vi "6812B_AC_old.vi"() -> ()   [LabVIEW 2019]
doc: "Shows how to generate a standard output."
uses:
  <instrlib>/Agilent 681x Series/Public/Data/Read Single Measurement (Current).vi
  <instrlib>/Agilent 681x Series/Agilent 681x Series.lvlib
panel:
  out "Flag":bool
  in  "Maximum Time (10000 ms)":i32=10000
  in  "Sense Source (0: Internal)":u16(ring) items=["Internal", "External"]
  in  "Sample Spacing (25 us)":dbl=2.5e-05 format="%^.2g"
  in  "Relative Trigger Samples (0)":i32
  out "Peak Current":dbl
  out "AC + DC RMS Current":dbl
  out "AC RMS Current":dbl
  out "DC Current":dbl
  in  "Pulse Characteristic Value (%)":dbl=50.0 format="%#.4g"
  in  "Pulse Characteristic (0: Duty Cycle)":u16(ring) items=["Duty Cycle", "Pulse Width"]
  in  "Period (s)":dbl=0.03333 format="%#.4g"
  in  "Trigger Delay (s)":dbl format="%#.5g"
  in  "Pulse Count":dbl=1.0 format="%#.4g"
  in  "Voltage Mode (0: Fix)":u16(ring) items=["Fixed", "Step", "Pulse", "List"]
  in  "Triggered Voltage Amplitude (V)":dbl=1.0 format="%#.4g"
  in  "Parar":bool
  in  "Peak Current Limit (13 A)":dbl=13.0 format="%#.4g"
  in  "RMS Current Limit (1 A)":dbl=1.0 format="%#.4g"
  in  "Voltage Amplitude (1.0 V)":dbl=1.0 format="%#.4g"
  in  "Output Frequency (60 Hz)":dbl=60.0 format="%#.4g"
  in  "Output Waveform Type (0: Sinusoid)":u16(ring) items=["Sinusoid", "Square", "Clipped Sinusoid", "User Specified"]
  in  "Serial Configuration":T1={"Baud Rate"=9600, "Parity"=0, "Data Bits"=8} {"Data Bits" items=["7"=7, "8"=8]; "Parity" items=["None", "Odd", "Even", "Mark", "Space"]; "Baud Rate" items=["300"=300, "600"=600, "1200"=1200, "2400"=2400, "4800"=4800, "9600"=9600]}
  in  "VISA resource name":refnum<visa-resource-name>
  # "(c) 2008-2021 National Instruments Corp.  ALL RIGHTS RESERVED."
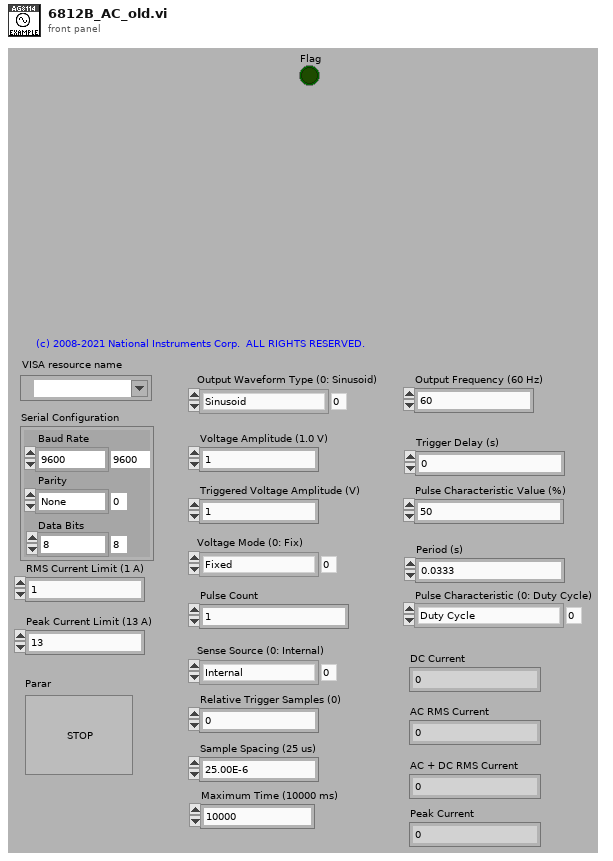
[diagram p1: front panel]
types:
  T1 = cluster{"Baud Rate":u32, "Parity":u16, "Data Bits":u16}
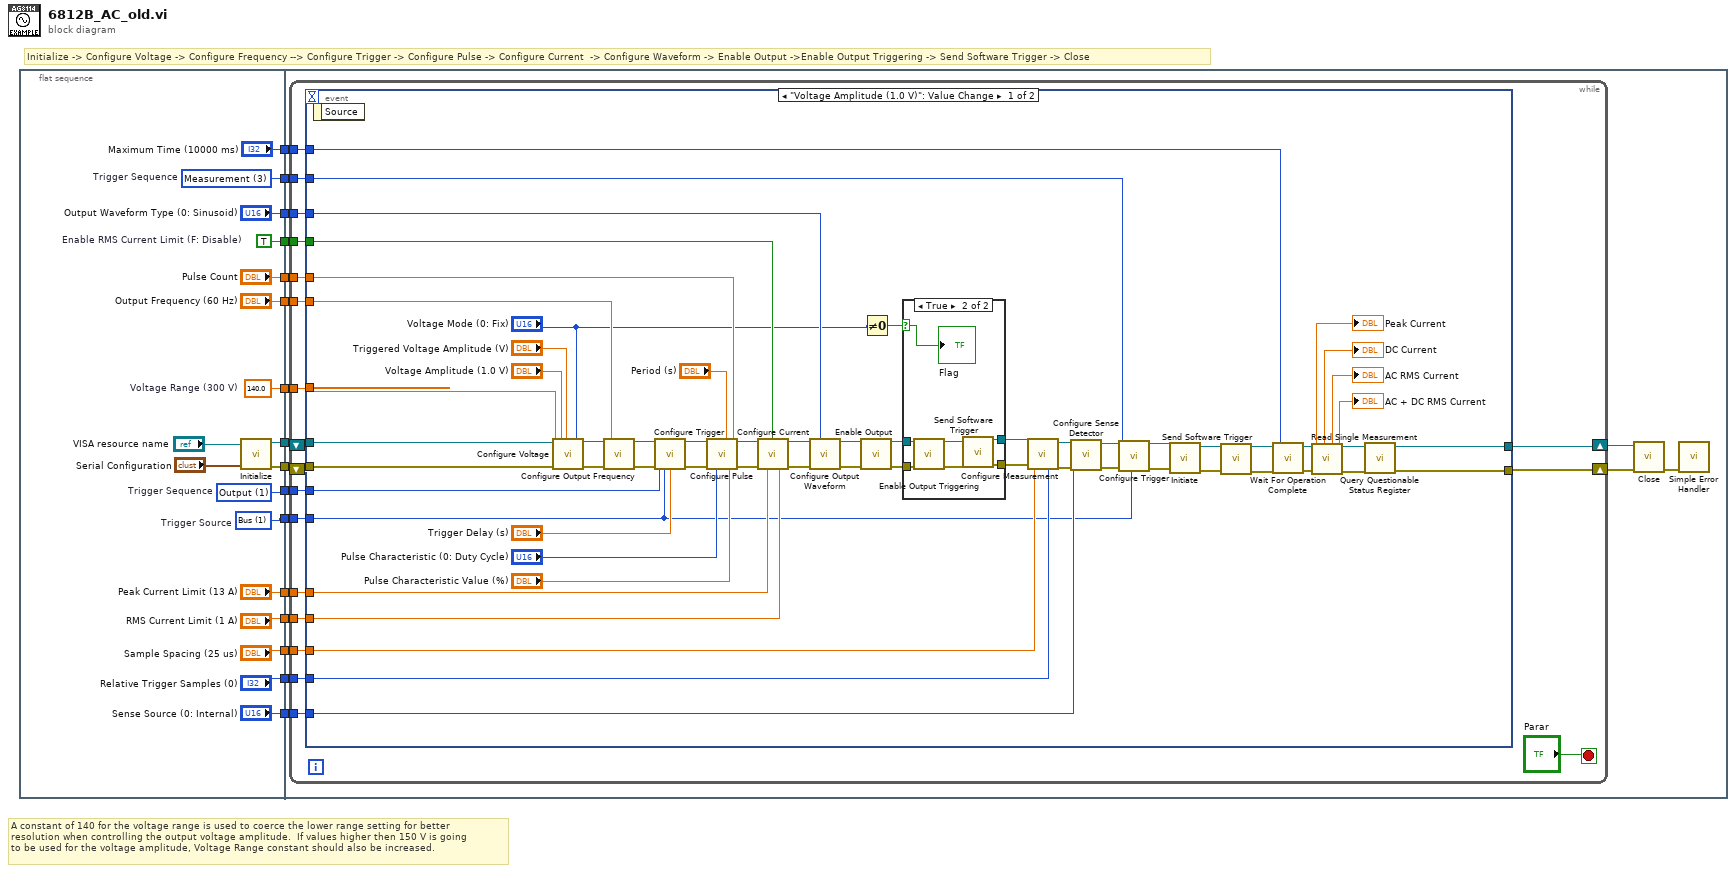
[diagram p0: block diagram]
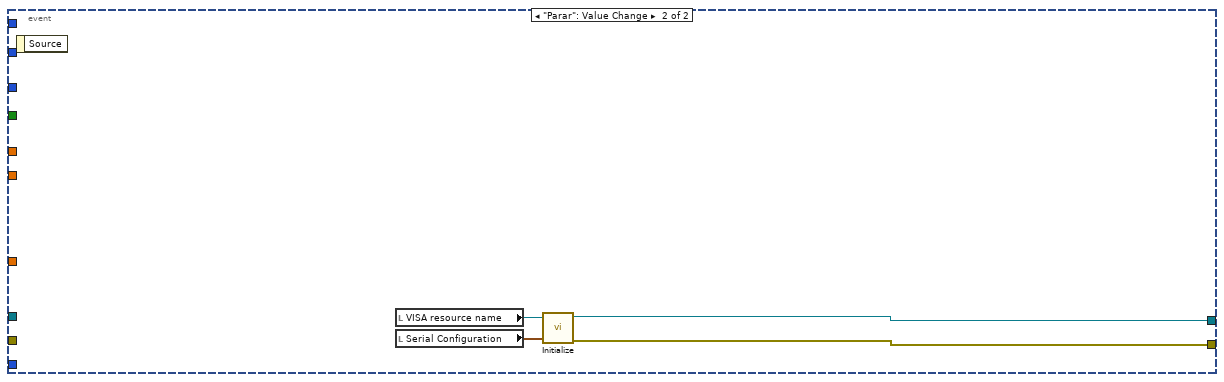
[diagram p3: hidden frame]
diagram:
  # "Initialize -> Configure Voltage -> Configure Frequency --> Configure Trigger -> Configure Pulse -> Configure Current  -> Configure Waveform -> Enable Output ->Enable Output Triggering -> Send Software Trigger -> Close"
  # "A constant of 140 for the voltage range is used to coerce the lower range setting for better\nresolution when controlling the output voltage amplitude.  If values higher then 150 V is going\nto be used for the voltage amplitude, Voltage Range constant should also be increased."
  n1 = flat-sequence {
    tunnel: [w34] -> w16
    tunnel: [w33] -> w15
    tunnel: ["Output Waveform Type (0: Sinusoid)"] -> w14
    tunnel: [w31] -> w13
    tunnel: [w30] -> w12
    tunnel: ["Output Frequency (60 Hz)"] -> w11
    tunnel: ["RMS Current Limit (1 A)"] -> w10
    tunnel: ["Peak Current Limit (13 A)"] -> w9
    tunnel: ["Pulse Count"] -> w8
    tunnel: [w23] -> w7
    tunnel: [w22] -> w6
    tunnel: ["Sense Source (0: Internal)"] -> w5
    tunnel: ["Sample Spacing (25 us)"] -> w4
    tunnel: ["Relative Trigger Samples (0)"] -> w3
    tunnel: [w18] -> w2
    tunnel: ["Maximum Time (10000 ms)"] -> w1
    tunnel: w16 -> [w50]
    tunnel: w15 -> [w49]
    tunnel: w14 -> [w48]
    tunnel: w13 -> [w47]
    tunnel: w12 -> [w46]
    tunnel: w11 -> [w45]
    tunnel: w10 -> [w44]
    tunnel: w9 -> [w43]
    tunnel: w8 -> [w42]
    tunnel: w7 -> [w41]
    tunnel: w6 -> [w40]
    tunnel: w5 -> [w39]
    tunnel: w4 -> [w38]
    tunnel: w3 -> [w37]
    tunnel: w2 -> [w36]
    tunnel: w1 -> [w35]
    frame #0 {
      w18 = 3 items=["Output"=1, "Synchronous Source"=2, "Measurement"=3]  # Trigger Sequence
      w22 = 1 items=["Immediate", "Bus", "External", "Phase", "Trigger Out"]  # Trigger Source
      w23 = 1 items=["Output"=1, "Synchronous Source"=2, "Measurement"=3]  # Trigger Sequence
      w30 = TRUE  # Enable RMS Current Limit (F: Disable)
      w31 = 140.0  # Voltage Range (300 V)
      n2 = call <instrlib>:"Initialize.vi"("Serial Configuration"="Serial Configuration", "VISA resource name"="VISA resource name") -> ("error out"=w33:errorcluster, "VISA resource name out"=w34:refnum<visa-resource-name>)  [unwired: 8 in]
    }
    frame #1 {
      n3 = while {
        tunnel: w48 -> [w68]
        tunnel: w47 -> [w67]
        tunnel: w46 -> [w66]
        tunnel: w45 -> [w65]
        tunnel: w44 -> [w64]
        tunnel: w43 -> [w63]
        shift-right: [w72] -> w52
        shift-left: w50 -> [w70]
        shift-right: [w71] -> w51
        shift-left: w49 -> [w69]
        tunnel: w42 -> [w62]
        tunnel: w41 -> [w61]
        tunnel: w40 -> [w60]
        tunnel: w39 -> [w59]
        tunnel: w38 -> [w58]
        tunnel: w37 -> [w57]
        tunnel: w36 -> [w56]
        tunnel: w35 -> [w55]
        stop <- "Parar" stop-if-true
        n4 = event shown="[0] \"Voltage Amplitude (1.0 V)\": Value Change" {
          selector: _ -> [_ _]
          dyn-events: _ -> [_ _]
          timeout: _ -> [_ _]
          tunnel: w70 -> [w103 _]
          tunnel: w69 -> [w102 _]
          tunnel: w68 -> [w132 _]
          tunnel: w67 -> [w131 _]
          tunnel: w66 -> [w128 _]
          tunnel: [w84 w145] -> w71
          tunnel: [w85 w144] -> w72
          tunnel: w65 -> [w122 _]
          tunnel: w64 -> [w127 _]
          tunnel: w63 -> [w126 _]
          tunnel: w62 -> [w113 _]
          tunnel: w61 -> [w109 _]
          tunnel: w60 -> [w79 _]
          tunnel: w59 -> [w106 _]
          tunnel: w58 -> [w105 _]
          tunnel: w57 -> [w104 _]
          tunnel: w56 -> [w83 _]
          tunnel: w55 -> [w82 _]
          event "Voltage Amplitude (1.0 V)": Value Change {
            n5 = event-data() -> ()  [unwired: 1 in, 1 out]
            n6 = call <instrlib>:"Configure Voltage.vi"("VISA resource name"=w103, "Triggered Voltage Amplitude (1.0 V)"="Triggered Voltage Amplitude (V)", "Voltage Range (300 V)"=w131, "Voltage Amplitude (1.0 V)"="Voltage Amplitude (1.0 V)", "Voltage Mode (0: Fix)"="Voltage Mode (0: Fix)", "error in (no error)"=w102) -> ("VISA resource name out"=w124:refnum<visa-resource-name>, "error out"=w123:errorcluster)  [unwired: 8 in]
            n7 = call <instrlib>:"Configure Output Frequency.vi"("VISA resource name"=w124, "Output Frequency (60 Hz)"=w122, "error in (no error)"=w123) -> ("VISA resource name out"=w121:refnum<visa-resource-name>, "error out"=w120:errorcluster)  [unwired: 11 in]
            n8 = call <instrlib>:"Configure Trigger.vi"("VISA resource name"=w121, "Trigger Sequence (1: Output 1)"=w109, "Trigger Source (0: Immediate)"=w79, "error in (no error)"=w120, "Trigger Delay (0 s)"="Trigger Delay (s)") -> ("VISA resource name out"=w119:refnum<visa-resource-name>, "error out"=w118:errorcluster)  [unwired: 9 in]
            n9 = call <instrlib>:"Configure Pulse.vi"("VISA resource name"=w119, "Pulse Count (1)"=w113, "Period (0.0333 s)"="Period (s)", "error in (no error)"=w118, "Pulse Characteristic (0: Duty Cycle)"="Pulse Characteristic (0: Duty Cycle)", "Pulse Characteristic Value (50)"="Pulse Characteristic Value (%)") -> ("VISA resource name out"=w117:refnum<visa-resource-name>, "error out"=w116:errorcluster)  [unwired: 8 in]
            n10 = call <instrlib>:"Configure Current.vi"("VISA resource name"=w117, "Enable RMS Current Limit (F: Disable)"=w128, "RMS Current Limit (1 A)"=w127, "error in (no error)"=w116, "Peak Current Limit (13 A)"=w126) -> ("VISA resource name out"=w115:refnum<visa-resource-name>, "error out"=w114:errorcluster)  [unwired: 9 in]
            n11 = call <instrlib>:"Configure Output Waveform.vi"("VISA resource name"=w115, "Output Waveform Type (0: Sinusoid)"=w132, "error in (no error)"=w114) -> ("VISA resource name out"=w129:refnum<visa-resource-name>, "error out"=w130:errorcluster)  [unwired: 11 in]
            n12 = call <instrlib>:"Enable Output.vi"("VISA resource name"=w129, "error in (no error)"=w130) -> ("VISA resource name out"=w78:refnum<visa-resource-name>, "error out"=w77:errorcluster)  [unwired: 12 in]
            n13 = Not Equal To 0?(x="Voltage Mode (0: Fix)") -> (x != 0?=w73:bool)
            n14 = case shown="True" w73 {
              selector: w73 -> [_ w135]
              tunnel: w78 -> [w134 w139]
              tunnel: w77 -> [w133 w138]
              tunnel: [w134 w137] -> w76
              tunnel: [w133 w136] -> w75
              frame False {
              }
              frame True {
                n15 = call <instrlib>:"Enable Output Triggering.vi"("VISA resource name"=w139, "error in (no error)"=w138) -> ("VISA resource name out"=w140:refnum<visa-resource-name>, "error out"=w141:errorcluster)  [unwired: 12 in]
                n16 = call <instrlib>:"Send Software Trigger.vi"("VISA resource name"=w140, "error in (no error)"=w141) -> ("VISA resource name out"=w137:refnum<visa-resource-name>, "error out"=w136:errorcluster)  [unwired: 12 in]
                "Flag" <- w135
              }
            }
            n17 = call <instrlib>:"Configure Measurement.vi"("VISA resource name"=w76, "Relative Trigger Samples (0)"=w104, "Sample Spacing (25 us)"=w105, "error in (no error)"=w75) -> ("VISA resource name out"=w101:refnum<visa-resource-name>, "error out"=w100:errorcluster)  [unwired: 10 in]
            n18 = call <instrlib>:"Configure Sense Detector.vi"("VISA resource name"=w101, "Sense Source (0: Internal)"=w106, "error in (no error)"=w100) -> ("VISA resource name out"=w81:refnum<visa-resource-name>, "error out"=w80:errorcluster)  [unwired: 11 in]
            n19 = call <instrlib>:"Configure Trigger.vi"("VISA resource name"=w81, "Trigger Sequence (1: Output 1)"=w83, "Trigger Source (0: Immediate)"=w79, "error in (no error)"=w80) -> ("VISA resource name out"=w94:refnum<visa-resource-name>, "error out"=w93:errorcluster)  [unwired: 10 in]
            n20 = call <instrlib>:"Initiate.vi"("error in (no error)"=w93, "VISA resource name"=w94) -> ("error out"=w92:errorcluster, "VISA resource name out"=w95:refnum<visa-resource-name>)  [unwired: 8 in]
            n21 = call <instrlib>:"Send Software Trigger.vi"("VISA resource name"=w95, "error in (no error)"=w92) -> ("VISA resource name out"=w91:refnum<visa-resource-name>, "error out"=w90:errorcluster)  [unwired: 12 in]
            n22 = call <instrlib>:"Wait For Operation Complete.vi"("error in (no error)"=w90, "Maximum Time (10000 ms)"=w82, "VISA resource name"=w91) -> ("error out"=w88:errorcluster, "VISA resource name out"=w89:refnum<visa-resource-name>)  [unwired: 7 in]
            n23 = call-poly <instrlib>:"Read Single Measurement.vi"("VISA resource name"=w89, "error in (no error)"=w88) -> ("Peak Current"=→"Peak Current":dbl, "VISA resource name out"=w87:refnum<visa-resource-name>, "DC Current"=→"DC Current":dbl, "AC RMS Current"=→"AC RMS Current":dbl, "AC + DC RMS Current"=→"AC + DC RMS Current":dbl, "error out"=w86:errorcluster)  [unwired: 8 in]
            n24 = call <instrlib>:"Query Questionable Status Register.vi"("error in (no error)"=w86, "VISA resource name"=w87) -> ("error out"=w84:errorcluster, "VISA resource name out"=w85:refnum<visa-resource-name>)  [unwired: 7 in, 1 out]
          }
          event "Parar": Value Change {
            n25 = event-data() -> ()  [unwired: 1 in, 1 out]
            n26 = local read "VISA resource name"() -> (w143:refnum<visa-resource-name>)
            n27 = local read "Serial Configuration"() -> (w142:T1)
            n28 = call <instrlib>:"Initialize.vi"("Serial Configuration"=w142, "VISA resource name"=w143) -> ("error out"=w145:errorcluster, "VISA resource name out"=w144:refnum<visa-resource-name>)  [unwired: 8 in]
          }
        }
      }
      n29 = call <instrlib>:"Close.vi"("error in (no error)"=w51, "VISA resource name"=w52) -> ("error out"=w53:errorcluster)  [unwired: 9 in]
      n30 = call <vilib>:"Simple Error Handler.vi"("error in (no error)"=w53) -> ()  [unwired: 4 in, 5 out]
    }
  }
